vi "string2boolen.vi"(1 "String":string) -> (0 "Boolean":bool)   [LabVIEW 2013]
doc: "此函数当且仅当字符串中包含字符‘1’时返回TRUE，否则返回FALSE"
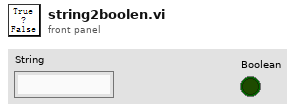
[diagram p1: front panel]
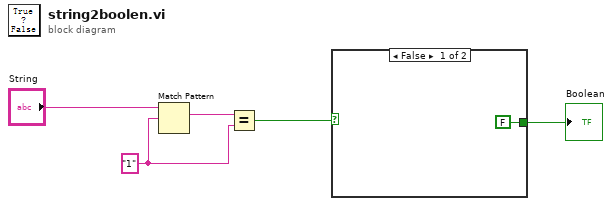
[diagram p0: block diagram]
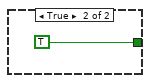
[diagram p2: hidden frame]
diagram:
  w3 = "1" ("regular expression")
  n1 = Match Pattern(string="String", regular expression=w3) -> (match substring=w4:string)  [unwired: 1 in, 3 out]
  n2 = Equal?(x=w4, y=w3) -> (x = y?=w2:bool)
  n3 = case shown="False" w2 {
    tunnel: [FALSE TRUE] -> w1
    frame False {
    }
    frame True {
    }
  }
  "Boolean" <- w1
